vi "random action.vi"(10 "Actions to choose from":T1[](array[typedef])) -> (2 "Action":T1)   [LabVIEW 2015, in "JFD_Common.lvlib"]
uses:
  JFD_Common.lvlib
  Type Defs/Action Enum.ctl
  Type Defs/SB Type Defs.lvlib
panel:
  in  "must move?":bool
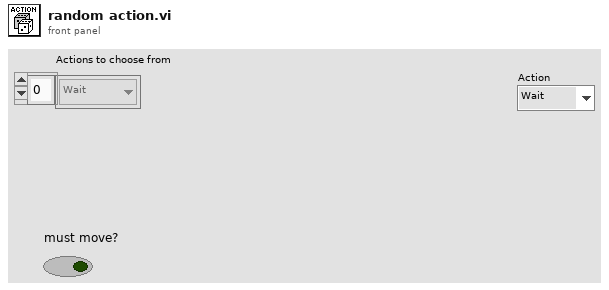
[diagram p1: front panel]
types:
  T1 = typedef "SB Type Defs.lvlib/Action Enum.ctl" = enum16{"Wait", "Move", "Attack", "Replicate"}
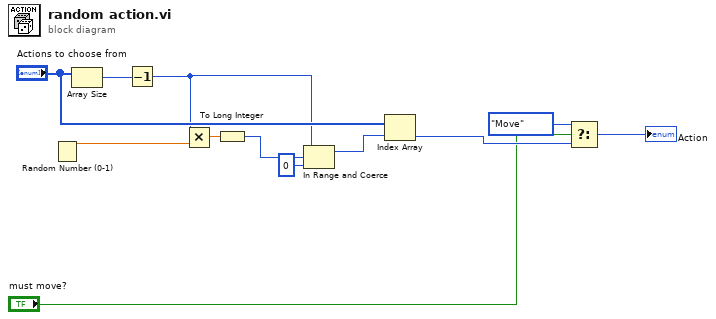
[diagram p0: block diagram]
diagram:
  n1 = Random Number (0-1)() -> (number: 0 to 1=w12:dbl)
  n2 = Array Size(array="Actions to choose from") -> (size(s)=w6:i32)
  n3 = Decrement(x=w6) -> (x-1=w5:i32)
  n4 = Multiply(x=w5, y=w12) -> (x*y=w11:dbl)
  n5 = To Long Integer(number=w11) -> (32bit integer=w8:i32)
  n6 = In Range and Coerce(upper limit=w5, x=w8, lower limit=0) -> (coerced(x)=w7:i32)  [unwired: 1 out]
  n7 = Index Array(array="Actions to choose from", index=w7) -> (element=w4:T1)
  n8 = Select(t=Action_Enum."Move", s="must move?", f=w4) -> (s? t:f=→"Action":T1)
